vi "SubPanel_DataCollection_Rev11_v5.vi"(0 "DCPowerInformationClusterArray_Input":T6(array[cluster]), 1 "VISAPowerInfoInputArray":T11(array[cluster]), 2 "Run Data SubPanel Input":T10, 3 "RF Block Parameters":T9, 4 "Oscilloscope Info Array":T8(array[cluster]) {"vertical coupling" items=["AC", "DC", "Ground"]}, 6 "New Run?":bool, 7 "error in":errorcluster) -> (10 "data iterating in loop":T2(array[cluster]), 12 "each channel cluster":T2(array[cluster]), 13 "Array of all channels?":dbl[][](array[numeric]), 14 "all channel clusters as a large array":T1(array[cluster]), 16 "data going into the binary file":T3, 20 "DCPowerInformationClusterArray_Output":T6(array[cluster]), 21 "VISAPowerInfoInputOutput":T11(array[cluster]), 22 "Run Data SubPanel Output":T10, 23 "RF Block Parameters Output":T9, 24 "Oscilloscope Info Array Output":T8(array[cluster]) {"vertical coupling" items=["AC", "DC", "Ground"]}, 25 "Reinitialize?":bool, 26 "Data Was Collected?":bool, 27 "error out":errorcluster)   [LabVIEW 2019]
uses:
  Controls/QueueDataControl.ctl
  Controls/DataBlockControl.ctl
  Controls/QueueDataControl_V2.ctl
  <vilib>/Analysis/NI_AALBase.lvlib
  Controls/QueueDataControl_V3.ctl
  <vilib>/Analysis/1siggen.llb/Ramp Pattern by Delta.vi
  <vilib>/Utility/file.llb/Write Delimited Spreadsheet (DBL).vi
  Controls/RFBlockControl.ctl
  <instrlib>/niScope/Controls/niScope vertical coupling.ctl
panel:
  out "supplemental datafile concatenated":i32[](array[numeric])
  out "supplemental datafile array":i32[][](array[numeric])
  out "supplemental datafile":i32[](array[numeric])
  out "datafile in array":T4[][](array[typedef])
  out "datafile in concatenation":T4[](array[typedef])
  out "datafile in loop":T4[](array[typedef])
  out "output cluster 2":T5
  out "Array":dbl[][][](array[numeric])
  out "DCPowerInformationClusterArray_Input 2":T6(array[cluster])
  out "Exiting":bool
  out "output cluster":T5
  out "Full Run Information":string
  out "Ready For Next Run?":bool
  in  "Next Run":bool
  out "Latchup Output Data":dbl[][](array[numeric])
  out "Recording Data":bool
  out "Current 2":waveform(dbl)[](graph)
  out "Voltage 2":waveform(dbl)[](graph)
  out "Current":waveform(dbl)[](graph)
  out "Voltage":waveform(dbl)[](graph)
  in  "End Collecting":bool
  in  "Record Data Toggle":bool
  out "error of collection":errorcluster
  in  "force exit SubVI":bool
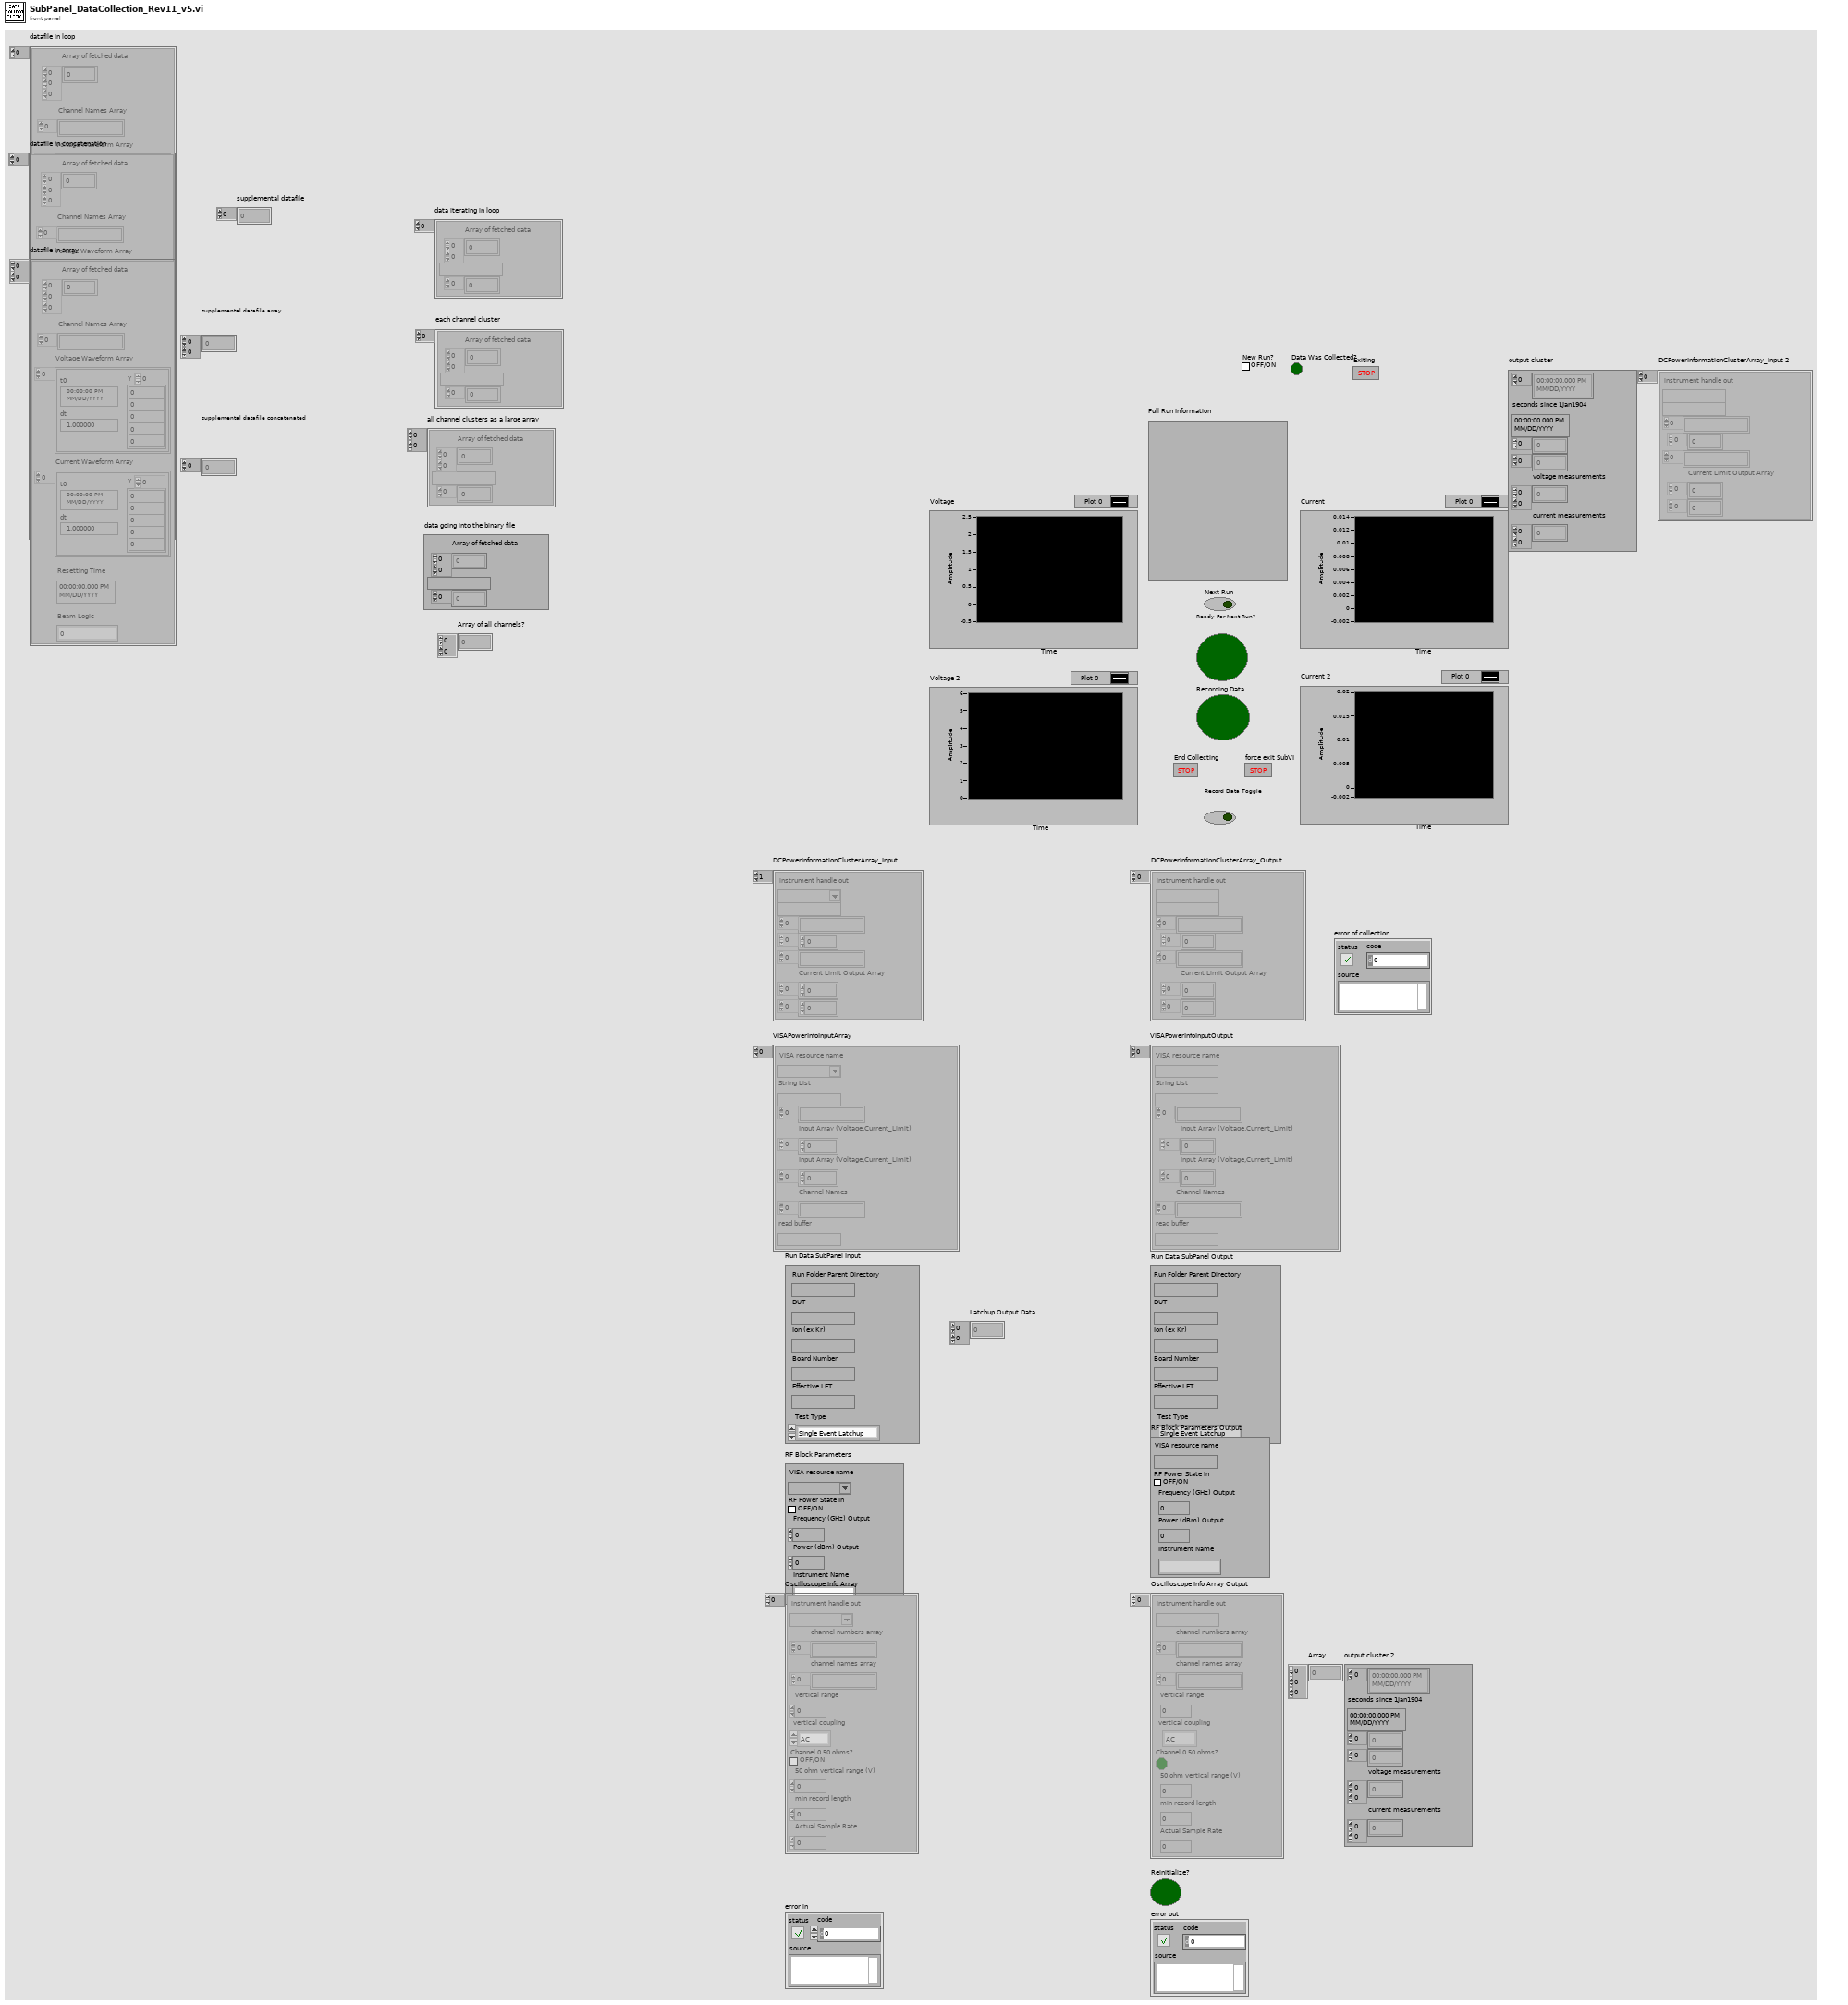
[diagram p1: front panel]
types:
  T1 = cluster{"Array of fetched data":dbl[][], string, i32[]}[][]
  T2 = cluster{"Array of fetched data":dbl[][], string, i32[]}[]
  T3 = cluster{"Array of fetched data":dbl[][], string, i32[]}
  T4 = typedef "QueueDataControl_V3.ctl" = cluster{"Array of fetched data":dbl[][][], "Channel Names Array":string[], "Voltage Waveform Array":waveform(dbl)[], "Current Waveform Array":waveform(dbl)[], "Resetting Time":timestamp, "Beam Logic":dbl}
  T5 = cluster{timestamp[], "seconds since 1Jan1904":timestamp, dbl[], i32[], "voltage measurements":dbl[][], "current measurements":dbl[][]}
  T6 = cluster{"instrument handle out":refnum<k15>, string, string[], dbl[], string[], "Current Limit Output Array":dbl[], dbl[]}[]
  T7 = typedef "niScope vertical coupling.ctl" = i32
  T8 = cluster{"instrument handle out":refnum<k15>, "channel numbers array":string[], "channel names array":string[], "vertical range":dbl, "vertical coupling":T7, "Channel 0 50 ohms?":bool, "50 ohm vertical range (V)":dbl, "min record length":i32, "Actual Sample Rate":dbl}[]
  T9 = typedef "RFBlockControl.ctl" = cluster{"VISA resource name":refnum<visa-resource-name>, "RF Power State In":bool, "Frequency (GHz) Output":dbl, "Power (dBm) Output":dbl, "Instrument Name":string}
  T10 = typedef "DataBlockControl.ctl" = cluster{"Run Folder Parent Directory":path, "DUT":string, "Ion (ex Kr)":string, "Board Number":string, "Effective LET":string, "Test Type":enum16{"Single Event Latchup", "Single Event Transient", "Single Event Upset"}}
  T11 = cluster{"VISA resource name":refnum<visa-resource-name>, "String List":string, string[], "Input Array (Voltage,Current_Limit)":dbl[], "Input Array (Voltage,Current_Limit)":dbl[], "Channel Names":string[], "read buffer":string}[]
  T12 = typedef "QueueDataControl_V2.ctl" = cluster{"Time Stamp Array":timestamp[], "Initial Time":timestamp, "dt measurement array":dbl[], "samples per capture":i32[], "voltage measurements":dbl[][], "current measurements":dbl[][]}
  T13 = cluster{"IVI Refnum out":refnum<k15>, string, "voltage level channel 23":dbl, "Channel Name 23":string, "Current Limit":dbl, "Measure Record dt":dbl, string, "Current Threshold Reset Value Array":dbl, "Mitigation Channel":bool}[]
  T14 = typedef "QueueDataControl.ctl" = cluster{"Rolling Timer":timestamp, "Initial Time":timestamp, "dt between samples":dbl[], "number of samples per fetch":i32[], "voltage measurements":dbl[][], "current measurements":dbl[][]}
  T15 = enum16{"big-endian, network order", "native, host order", "little-endian"}
  T16 = enum16{"open", "replace", "create", "open or create", "replace or create", "replace or create with confirmation"}
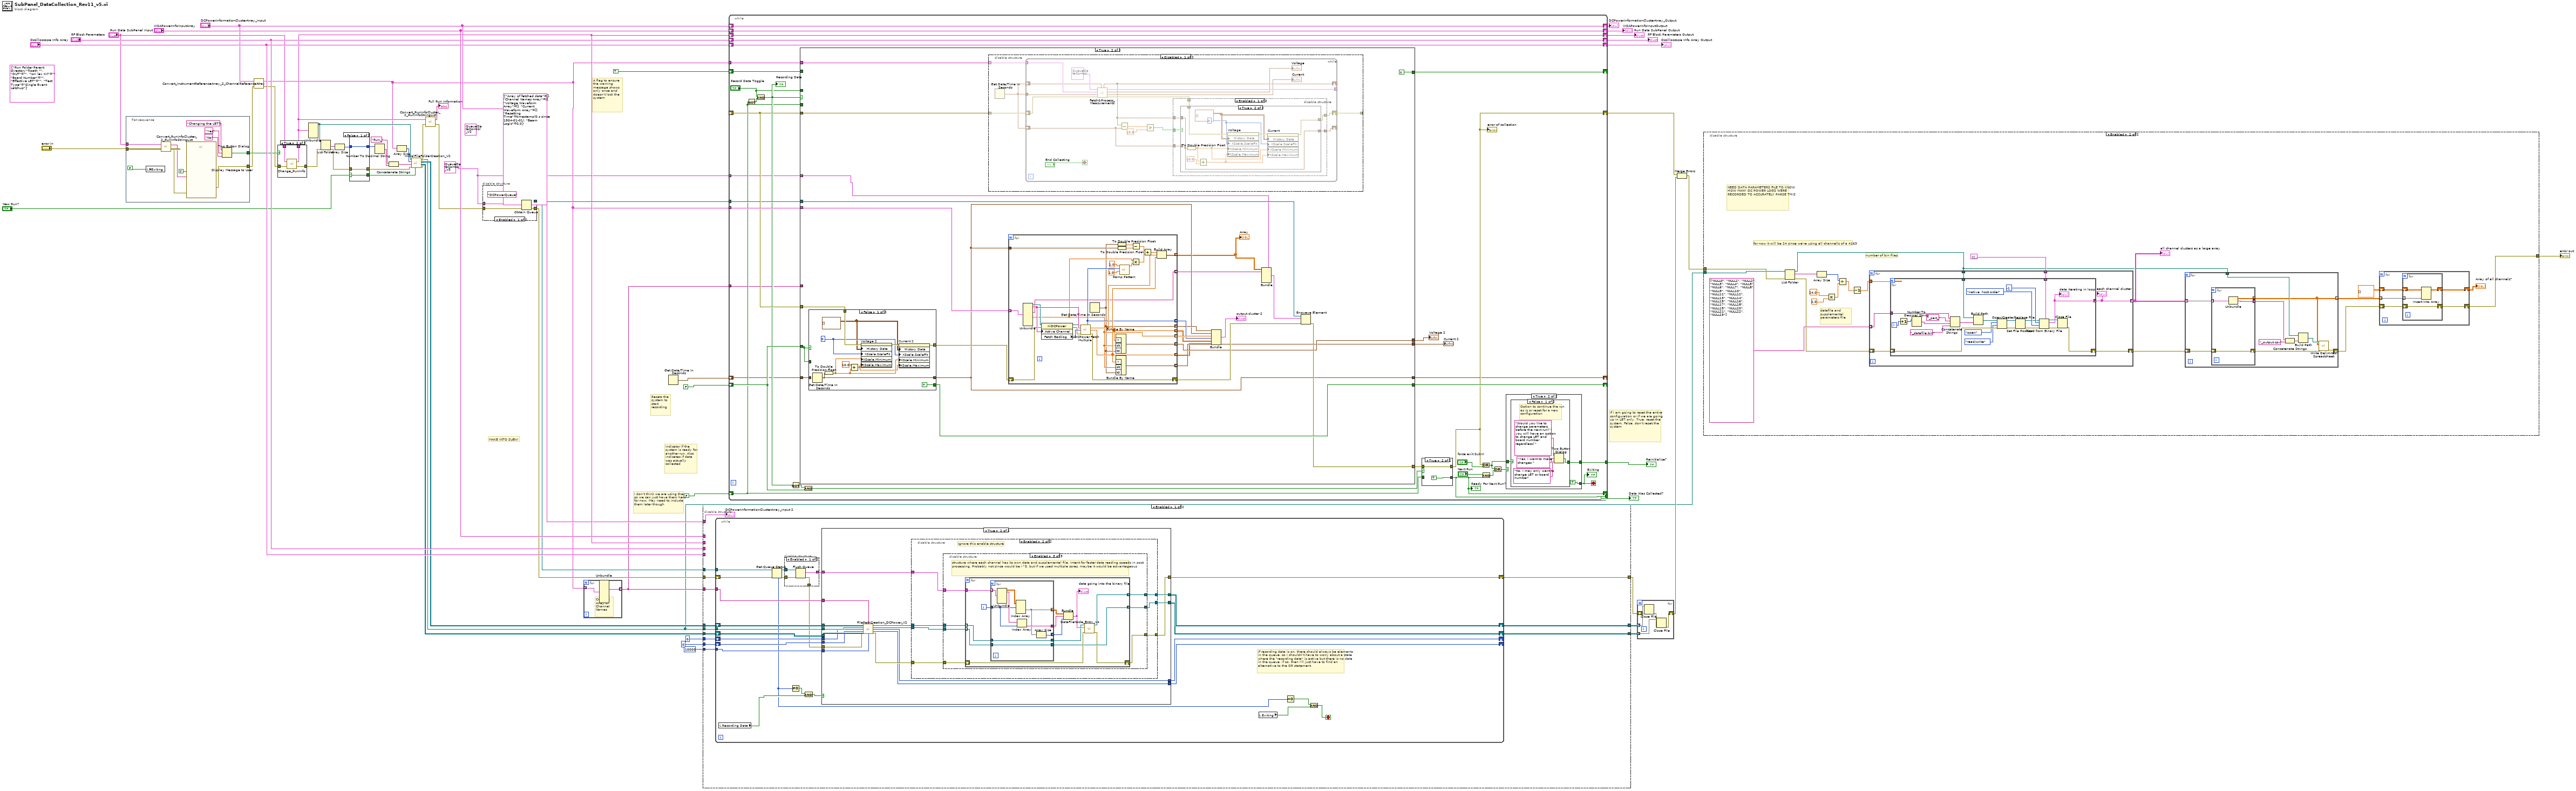
[diagram p0: block diagram]
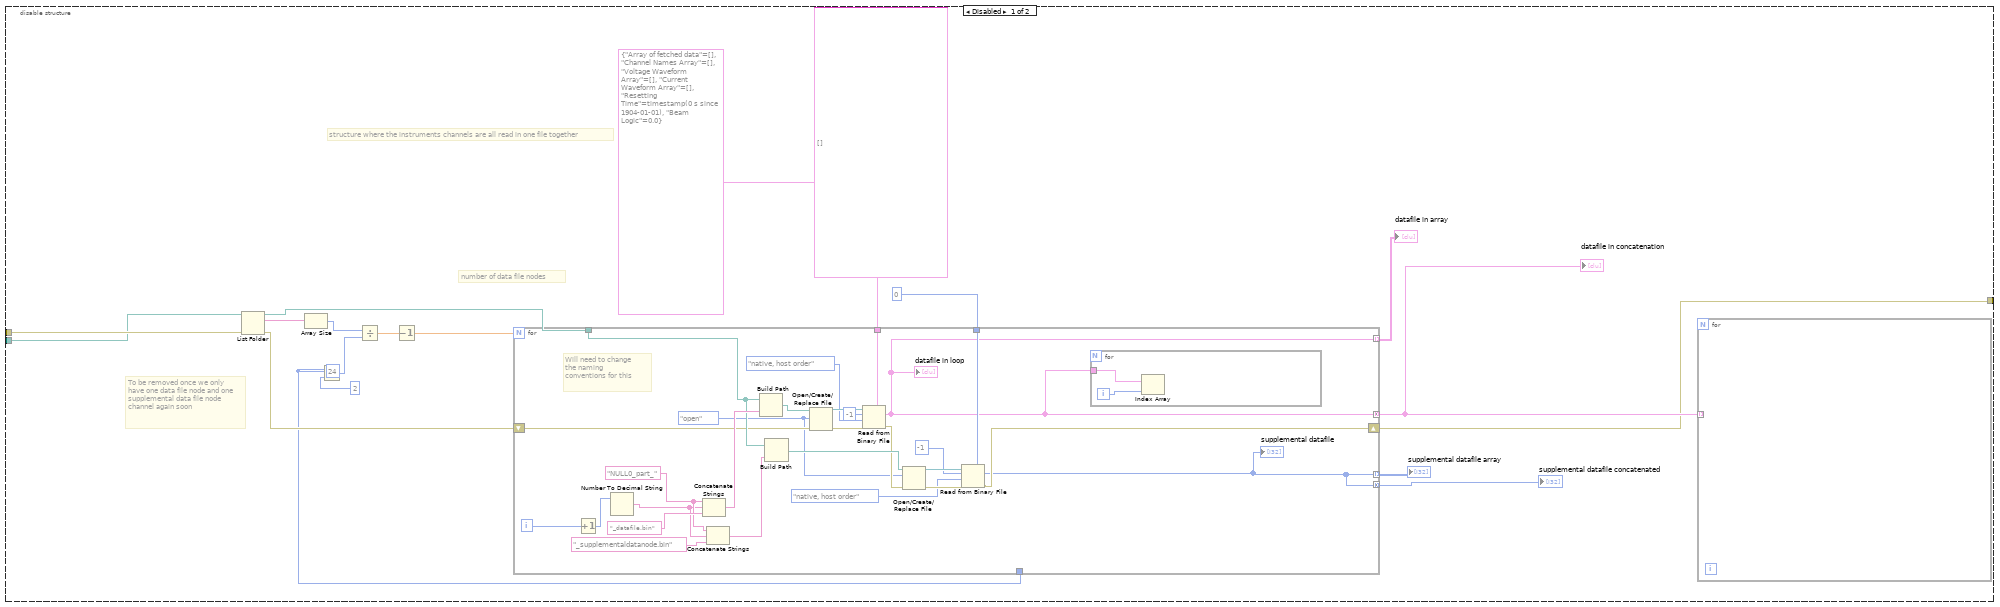
[diagram p2: hidden frame]
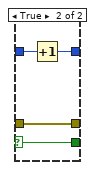
[diagram p3: hidden frame]
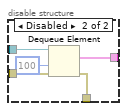
[diagram p6: hidden frame]
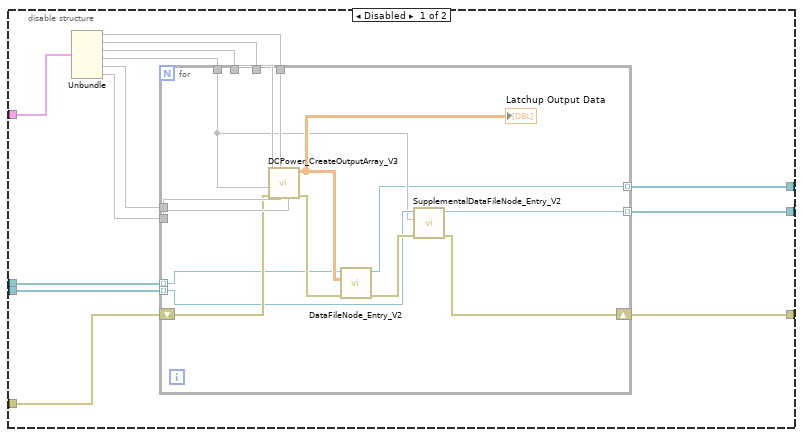
[diagram p8: hidden frame]
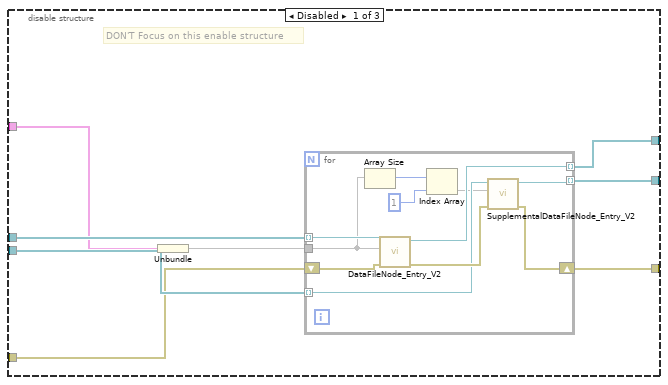
[diagram p9: hidden frame]
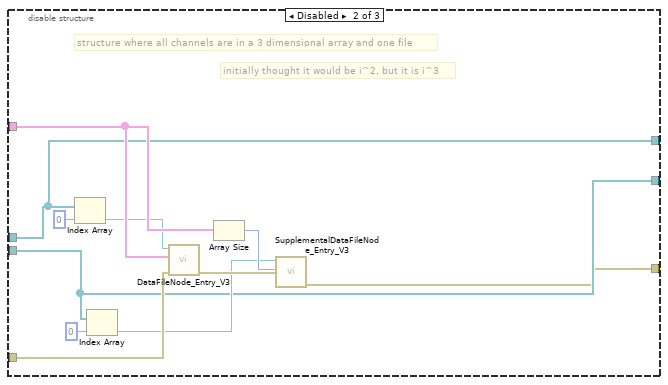
[diagram p10: hidden frame]
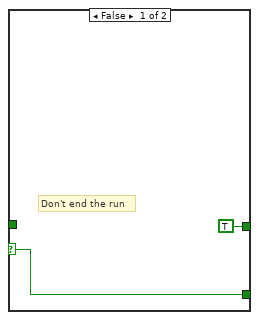
[diagram p12: hidden frame]
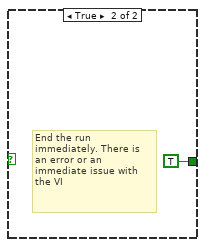
[diagram p13: hidden frame]
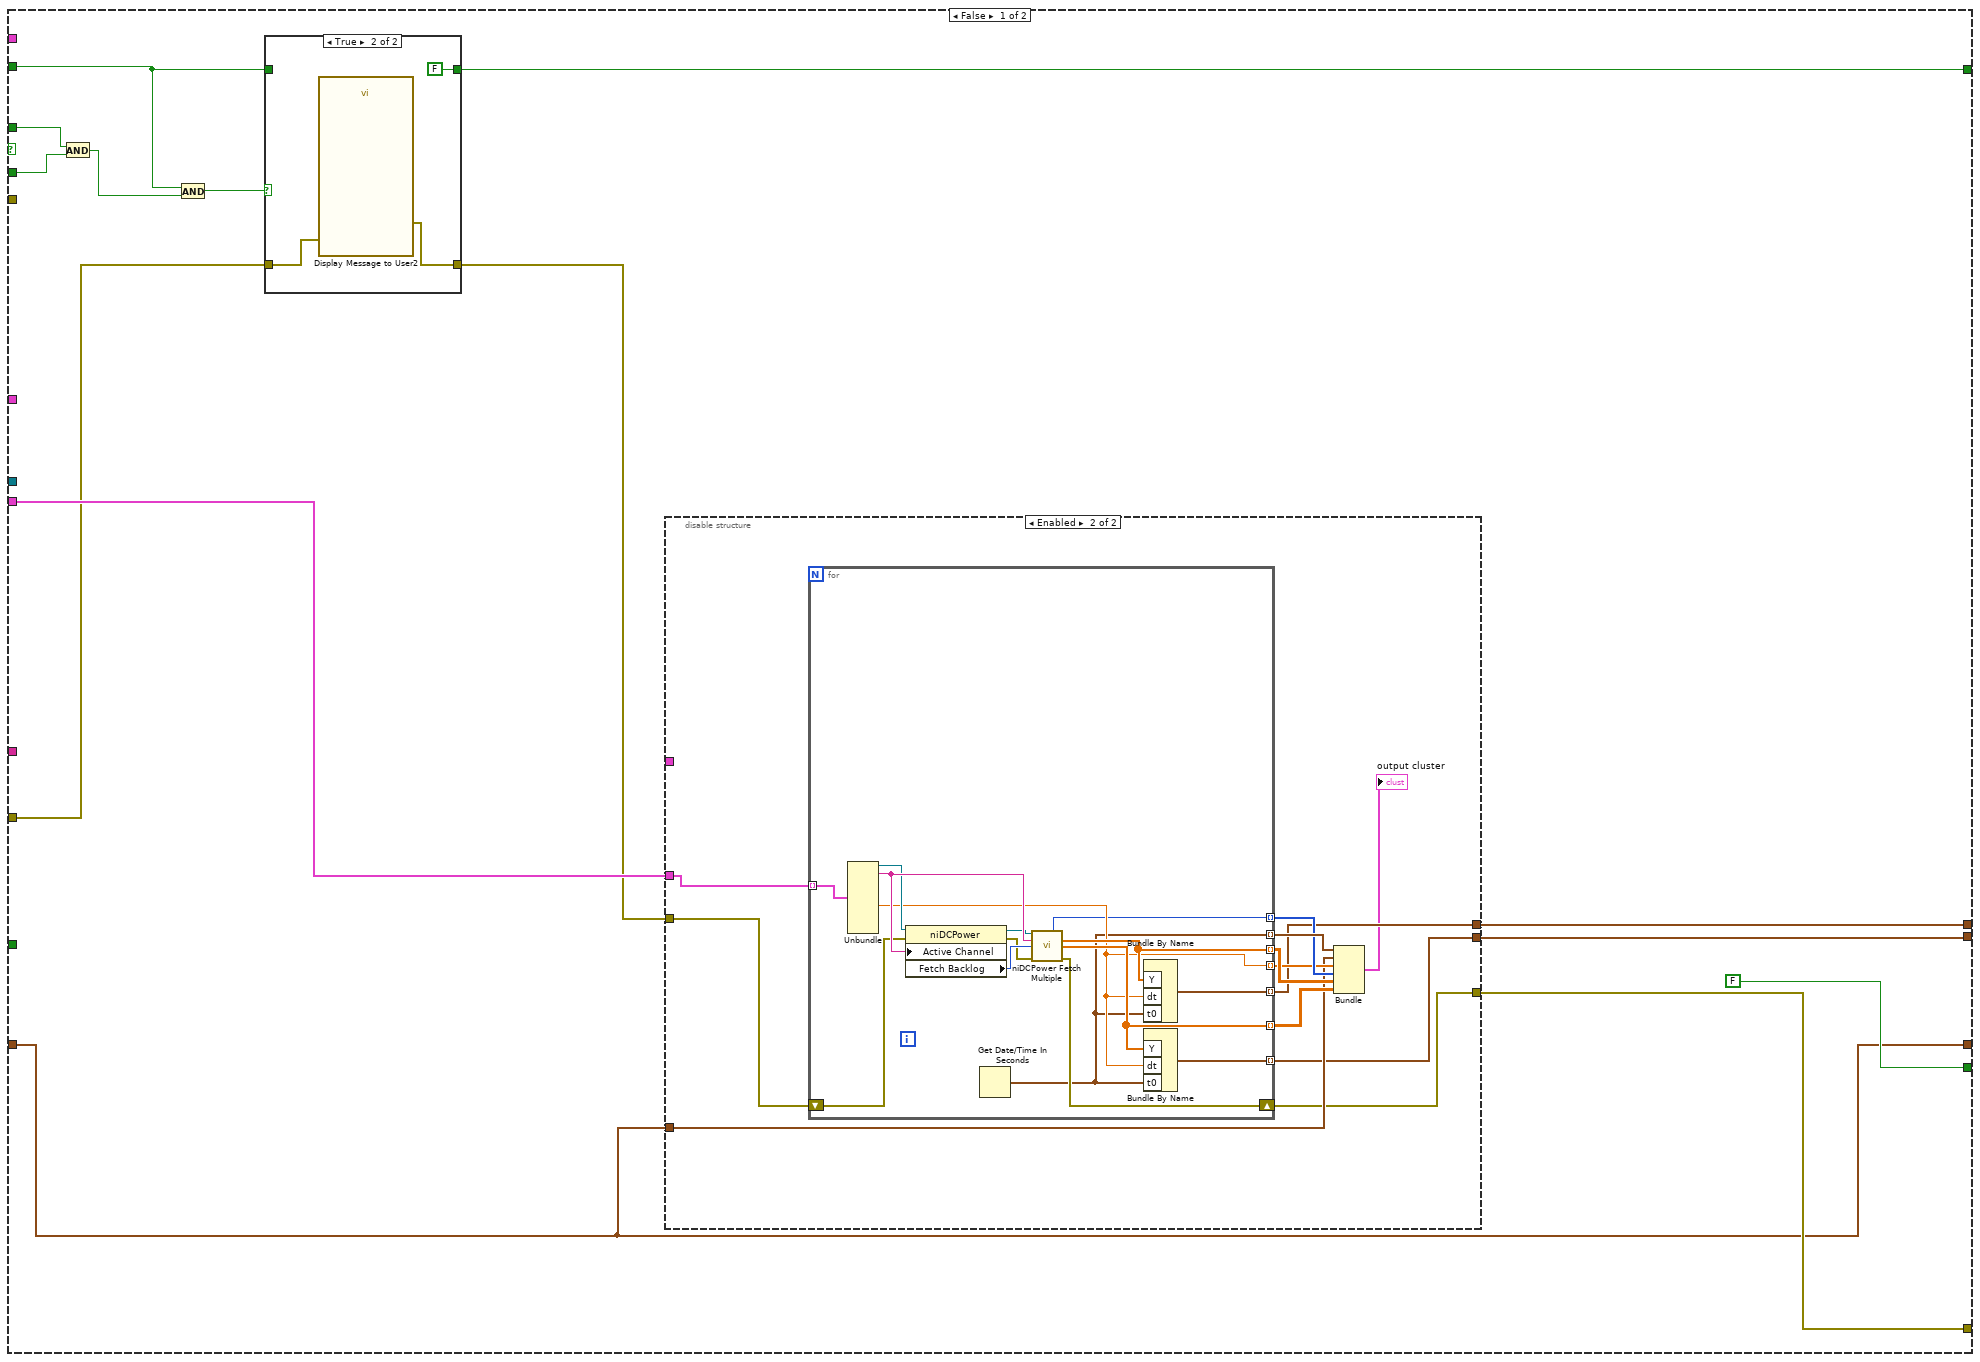
[diagram p15: hidden frame]
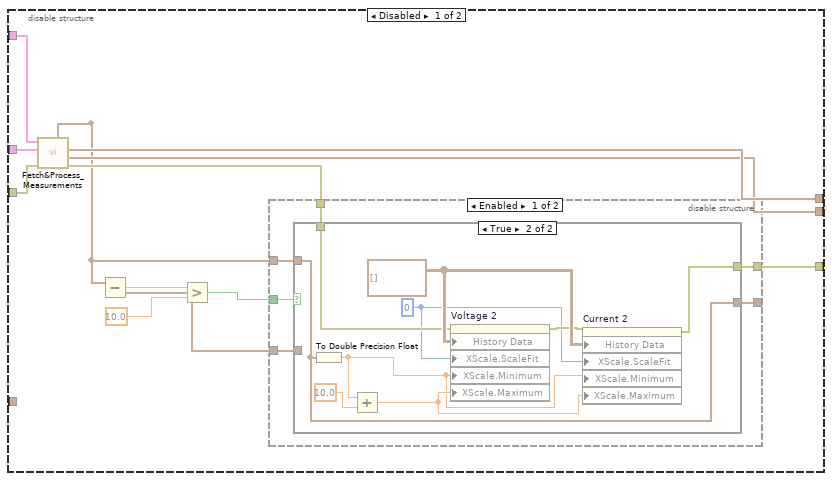
[diagram p16: hidden frame]
diagram:
  w8 = T4 {"Array of fetched data"=[], "Channel Names Array"=[], "Voltage Waveform Array"=[], "Current Waveform Array"=[], "Resetting Time"=timestamp(0 s since 1904-01-01), "Beam Logic"=0.0} ("DCPower Queue Data Double Array Format")
  (unwired) T4 {"Array of fetched data"=[], "Channel Names Array"=[], "Voltage Waveform Array"=[], "Current Waveform Array"=[], "Resetting Time"=timestamp(0 s since 1904-01-01), "Beam Logic"=0.0} ("DCPower Double Array Queue")
  (unwired) T12 {"Time Stamp Array"=[], "Initial Time"=timestamp(0 s since 1904-01-01), "dt measurement array"=[], "samples per capture"=[], "voltage measurements"=[], "current measurements"=[]} ("DCPowerDataQueueControl_V2")
  (unwired) T10 {"Run Folder Parent Directory"=path "", "DUT"="", "Ion (ex Kr)"="", "Board Number"="", "Effective LET"="", "Test Type"=enum."Single Event Latchup"} ("Run Data Configuration")
  # "I don't think we are using these so we can just have them here for now. May need to include them later though"
  # "Indicator if the system is ready for another run. Also indicates if data was actually collected"
  # "Resets the system to start recording"
  # "A flag to ensure the warning message shows only once and doesn't lock the system"
  # "If I am going to reset the entire configuration or if we are going up in LET only. True, reset the system. False, don't reset the system"
  # "MAKE INTO SUBVI"
  n1 = flat-sequence {
    tunnel: [w62] -> w31
    tunnel: "error in" -> [w61]
    tunnel: [w66] -> w40
    tunnel: "Run Data SubPanel Input" -> [w59]
    frame #0 {
      n2 = local write "Exiting"(FALSE ("Forced Exit")) -> ()
      n3 = call "Convert_RunInfoCluster_2_RunInfoStringList.vi"("error in"=w61, "Run Data SubPanel Input"=w59) -> ("error output"=w60:errorcluster, "Run Data Output"=w58:string)
      n4 = call "Display Message to User"("error in (no error)"=w60, "Enable"=TRUE, "Message"=w58) -> ("error out"=w62:errorcluster)  [unwired: 7 in, 1 out]
      n5 = Two Button Dialog(message="Changing the LET?", 1:"No" ("F button name (\"Cancel\")"), 2:"Yes" ("T button name (\"OK\")")) -> (T button?=w66:bool)
    }
  }
  n6 = call "Convert_InstrumentReferenceArray_2_ChannelReferenceArray.vi"("error in (no error)"=w31, "DCPowerInformationClusterArray_Input"="DCPowerInformationClusterArray_Input") -> ("error out"=w29:errorcluster, "DCPowerInformationArrayOutput_byChannel"=w14:T13)
  n7 = case shown="True" w40 {
    tunnel: "Run Data SubPanel Input" -> [w68 w72]
    tunnel: [w68 w71] -> w36
    tunnel: [w67 w70] -> w33
    tunnel: w29 -> [w67 w69]
    frame False {
    }
    frame True {
      n8 = call "Change_RunInfo.vi"("error in (no error)"=w69, "Run Data SubPanel in"=w72) -> ("error out"=w70:errorcluster, "Run Data SubPanel out"=w71:T10)
    }
  }
  n9 = Unbundle(w36) -> ("Run Folder Parent Directory"=w34:path)  [unwired: 5 out]
  n10 = List Folder(path=w34, error in=w33) -> (folder names=w35:string[], error out=w15:errorcluster)  [unwired: 2 in, 2 out]
  n11 = Array Size(array=w35) -> (size(s)=w18:i32)
  n12 = case shown="False" "New Run?" {
    selector: "New Run?" -> [w74 w77]
    tunnel: [w75 w79] -> w19
    tunnel: w18 -> [w75 w78]
    tunnel: [w74 w77] -> w17
    tunnel: [w73 w76] -> w16
    tunnel: w15 -> [w73 w76]
    frame False {
    }
    frame True {
      n13 = Increment(x=w78) -> (x+1=w79:i32)
    }
  }
  n14 = Number To Decimal String(number=w19) -> (decimal integer string=w23:string)  [unwired: 1 in]
  n15 = Concatenate Strings("Run_", w23) -> (w32:string)
  n16 = Array Size(array=w14) -> (size(s)=w13:i32)
  n17 = call "InitialFileFolderCreation_V2.vi"("New Run?"=w17, "error in (no error)"=w16, "Run Number"=w32, "Subfolders&NumChannelsRecorded"=w13, "base path"=w34) -> ("error out"=w12:errorcluster, "SupplementalDataFileReferenceObjectArrayWsubfolders"=w27:refnum<file>[][], "DataFileReferenceObjectArrayWsubfolders"=w28:refnum<file>[][], "created path array"=w2:path[])  [unwired: 3 in]
  n18 = call "Convert_RunInfoCluster_2_RunInfoStringList.vi"("error in"=w12, "Run Data SubPanel Input"=w36) -> ("error output"=w11:errorcluster, "Run Data Output"=→"Full Run Information":string)
  n19 = disable-structure shown="Enabled" {
    disable-tunnel: w11 -> [w83 w85]
    disable-tunnel: [w82 w85] -> w45
    disable-tunnel: [w81 _] -> w46
    disable-tunnel: w8 -> [w80 _]
    frame Enabled {
      n20 = Obtain Queue(name (unnamed)="DCPowerQueue", element data type=w80, error in (no error)=w83) -> (queue out=w81:refnum<queue>, error out=w82:errorcluster)  [unwired: 2 in, 1 out]
    }
    frame Disabled {
    }
  }
  n21 = for {
    tunnel: w14 -> [w87] mode=indexing
    tunnel: [w86] -> w9 mode=indexing
    # "Creating Array of Channel Names"
    n22 = Unbundle(w87) -> ("Channel Name 23"=w86:string)  [unwired: 8 out]
  }
  n23 = Get Date/Time In Seconds() -> (seconds since 1Jan1904=w37:timestamp)
  n24 = disable-structure shown="Enabled" {
    disable-tunnel: "DCPowerInformationClusterArray_Input" -> [w91 _]
    disable-tunnel: "VISAPowerInfoInputArray" -> [_ _]
    disable-tunnel: w36 -> [_ _]
    disable-tunnel: "RF Block Parameters" -> [_ _]
    disable-tunnel: "Oscilloscope Info Array" -> [_ _]
    disable-tunnel: w46 -> [w100 _]
    disable-tunnel: w45 -> [w99 _]
    disable-tunnel: w9 -> [w98 _]
    disable-tunnel: w2 -> [w97 _]
    disable-tunnel: w28 -> [w96 _]
    disable-tunnel: w27 -> [w95 _]
    disable-tunnel: 0 ("binary file indexor in") -> [w94 _]
    disable-tunnel: 0 ("binary file indexor in") -> [w93 _]
    disable-tunnel: 10000 ("binary file indexor in") -> [w92 _]
    disable-tunnel: [w90 _] -> w5
    disable-tunnel: [w89 _] -> w7
    disable-tunnel: [w88 _] -> w6
    frame Enabled {
      n25 = while {
        tunnel: w100 -> [w125]
        shift-right: [w112] -> w90
        shift-left: w99 -> [w124]
        tunnel: w97 -> [w121]
        shift-right: [w114] -> w89
        shift-left: w96 -> [w122]
        shift-right: [w113] -> w88
        shift-left: w95 -> [w120]
        shift-right: [w116] -> _
        shift-left: w94 -> [w119]
        shift-right: [w115] -> _
        shift-left: w93 -> [w118]
        tunnel: w92 -> [w117]
        tunnel: w98 -> [w123]
        stop <- w109 stop-if-true
        # "If recording data is on, there should always be elements in the queue, so I shouldn't have to worry about a state where the \"recording data\" is active but there is no data in the queue, if so, then I'll just have to find an alternative to the OR statement"
        n26 = local read "Recording Data"() -> (w102:bool)
        n27 = Get Queue Status(queue=w125, error in (no error)=w124) -> (queue out=w106:refnum<queue>, error out=w107:errorcluster, # elements in queue=w101:i32)  [unwired: 1 in, 5 out]
        n28 = disable-structure shown="Enabled" {
          disable-tunnel: [w129 w131] -> w108
          disable-tunnel: w107 -> [w128 w133]
          disable-tunnel: w106 -> [w127 w134]
          disable-tunnel: [w126 w130] -> w105
          frame Enabled {
            n29 = Flush Queue(queue=w127, error in (no error)=w128) -> (remaining elements=w126:T4[], error out=w129:errorcluster)  [unwired: 1 out]
          }
          frame Disabled {
            n30 = Dequeue Element(queue=w134, timeout in ms (-1)=100, error in (no error)=w133) -> (element=w130:T4, error out=w131:errorcluster)  [unwired: 2 out]
          }
        }
        n31 = Not Equal To 0?(x=w101) -> (x != 0?=w104:bool)
        n32 = And(x=w104, y=w102) -> (x .and. y?=w103:bool)
        n33 = case shown="True" w103 {
          tunnel: w105 -> [_ w156]
          tunnel: w108 -> [w137 w149]
          tunnel: w123 -> [_ w155]
          tunnel: w122 -> [w138 w154]
          tunnel: w121 -> [_ w153]
          tunnel: w120 -> [w139 w152]
          tunnel: w119 -> [w136 w151]
          tunnel: w118 -> [w135 w148]
          tunnel: w117 -> [_ w147]
          tunnel: [w136 w146] -> w116
          tunnel: [w135 w145] -> w115
          tunnel: [w138 w142] -> w114
          tunnel: [w139 w141] -> w113
          tunnel: [w137 w140] -> w112
          frame False {
          }
          frame True {
            n34 = call "FilePathCreation_DCPower_V2.vi"("binary file input reference array 1"=w154, "Channel Name Input array"=w155, "data output directory folder"=w153, "binary file indexor in"=w151, "Reset counter in"=w148, "error in (no error)"=w149, "binary file input reference array 2"=w152, "reset threshold"=w147) -> ("binary file output reference array"=w144:refnum<file>[], "binary file output reference array 2"=w143:refnum<file>[], "binary file indexor out"=w146:i32, "reset counter out"=w145:i32, "error out"=w150:errorcluster)  [unwired: 3 in]
            n35 = disable-structure shown="Enabled" {
              disable-tunnel: w156 -> [w169 w185]
              disable-tunnel: w150 -> [w168 w189]
              disable-tunnel: w144 -> [w167 w191]
              disable-tunnel: w143 -> [w166 w190]
              disable-tunnel: [w165 w188] -> w142
              disable-tunnel: [w164 w187] -> w141
              disable-tunnel: [w163 w186] -> w140
              frame Disabled {
                n36 = Unbundle(w169) -> (w157, w158, w162, w161, w160, w159)
                n37 = for {
                  tunnel: w162 -> [w182]
                  tunnel: w161 -> [w172]
                  tunnel: w160 -> [w181]
                  tunnel: w159 -> [w180]
                  tunnel: w158 -> [w183]
                  tunnel: w157 -> [w184]
                  shift-right: [w174] -> w163
                  shift-left: w168 -> [w179]
                  tunnel: w167 -> [w176] mode=indexing
                  tunnel: w166 -> [w173] mode=indexing
                  tunnel: [w171] -> w165 mode=indexing
                  tunnel: [w170] -> w164 mode=indexing
                  n38 = call "DCPower_CreateOutputArray_V3.vi"("current measurements"=w180, "voltage measurements"=w181, "Time Stamp Array"=w184, "error in"=w179, "actual count"=w172, "Measure Record dt"=w182, "Initial Time"=w183) -> ("error out"=w178:errorcluster, "Data Output Array"=w177:dbl[][])  [unwired: 3 in]
                  "Latchup Output Data" <- w177
                  n39 = call "DataFileNode_Entry_V2.vi"("error in (no error)"=w178, "Data Output Array"=w177, "Byte Stream File in"=w176) -> ("error out"=w175:errorcluster, "Byte Stream File out"=w171:refnum<file>)  [unwired: 7 in]
                  n40 = call "SupplementalDataFileNode_Entry_V2.vi"("error in (no error)"=w175, "actual count"=w172, "Byte Stream File in"=w173) -> ("error out"=w174:errorcluster, "Byte Stream File out"=w170:refnum<file>)  [unwired: 7 in]
                }
              }
              frame Enabled {
                # "Ignore this enable structure"
                n41 = disable-structure shown="Enabled" {
                  disable-tunnel: w191 -> [w199 w213 w228]
                  disable-tunnel: w190 -> [w198 w212 w227]
                  disable-tunnel: w189 -> [w197 w221 w225]
                  disable-tunnel: [w196 w213 w223] -> w188
                  disable-tunnel: [w195 w212 w222] -> w187
                  disable-tunnel: [w194 w211 w226] -> w186
                  disable-tunnel: w185 -> [w193 w218 w224]
                  frame Disabled {
                    # "DON'T Focus on this enable structure"
                    n42 = Unbundle(w193) -> (w192)
                    n43 = for {
                      tunnel: w192 -> [w207]
                      tunnel: w199 -> [w209] mode=indexing
                      tunnel: w198 -> [w208] mode=indexing
                      tunnel: [w205] -> w196 mode=indexing
                      tunnel: [w204] -> w195 mode=indexing
                      shift-right: [w203] -> w194
                      shift-left: w197 -> [w206]
                      n44 = Array Size(array=w207) -> (size(s)=w202:i32)
                      n45 = call "DataFileNode_Entry_V2.vi"("error in (no error)"=w206, "Data Output Array"=w207, "Byte Stream File in"=w209) -> ("error out"=w210:errorcluster, "Byte Stream File out"=w205:refnum<file>)  [unwired: 7 in]
                      n46 = Index Array(array=w202, index=1) -> (element=w200)
                      n47 = call "SupplementalDataFileNode_Entry_V2.vi"("error in (no error)"=w210, "actual count"=w200, "Byte Stream File in"=w208) -> ("error out"=w203:errorcluster, "Byte Stream File out"=w204:refnum<file>)  [unwired: 7 in]
                    }
                  }
                  frame Disabled {
                    # "initially thought it would be i^2, but it is i^3"
                    # "structure where all channels are in a 3 dimensional array and one file"
                    n48 = Index Array(array=w213, index=0) -> (element=w214:refnum<file>)
                    n49 = Index Array(array=w212, index=0) -> (element=w215:refnum<file>)
                    n50 = call "DataFileNode_Entry_V3.vi"("error in (no error)"=w221, "remaining elements"=w218, "Byte Stream File in"=w214) -> ("error out"=w220:errorcluster)  [unwired: 7 in, 1 out]
                    n51 = Array Size(array=w218) -> (size(s)=w219:i32)
                    n52 = call "SupplementalDataFileNode_Entry_V3.vi"("error in (no error)"=w220, "actual count"=w219, "Byte Stream File in"=w215) -> ("error out"=w211:errorcluster)  [unwired: 7 in, 1 out]
                  }
                  frame Enabled {
                    # "structure where each channel has its own data and supplemental file. Intent for faster data reading speeds in post processing. Probably not since would be i^3, but if we used multiple cores, maybe it would be advantageous"
                    n53 = for {
                      tunnel: w228 -> [w236] mode=indexing
                      tunnel: w227 -> [w237] mode=indexing
                      shift-right: [w229] -> w226
                      shift-left: w225 -> [w232]
                      tunnel: w224 -> [w241]
                      tunnel: [w231] -> w223 mode=indexing
                      tunnel: [w230] -> w222 mode=indexing
                      i -> [w240]
                      n54 = for {
                        tunnel: w241 -> [w250] mode=indexing
                        tunnel: w240 -> [w247]
                        tunnel: [w243] -> w239 mode=concatenating
                        tunnel: [w246] -> w238
                        tunnel: w237 -> [w244]
                        tunnel: w236 -> [w245]
                        tunnel: [w245] -> w233
                        tunnel: [w244] -> w230
                        tunnel: [w242] -> w235 mode=concatenating
                        n55 = Unbundle(w250) -> ("Array of fetched data"=w249:dbl[][][], "Channel Names Array"=w248:string[])  [unwired: 4 out]
                        n56 = Index Array(array=w249, index (dim 0)=w247) -> (element=w243:dbl[][])  [unwired: 2 in]
                        n57 = Index Array(array=w248, index=w247) -> (element=w246:string)
                        n58 = Array Size(array=w243) -> (size(s)=w242:i32[])
                      }
                      n59 = Bundle("Array of fetched data"=w239, w238, w235) -> (w234:T3)  [unwired: 1 in]
                      "data going into the binary file" <- w234
                      n60 = call "DataFileNode_Entry_V4.vi"("error in (no error)"=w232, "Queued Elements"=w234, "Byte Stream File in"=w233) -> ("error out"=w229:errorcluster, "Byte Stream File out"=w231:refnum<file>)  [unwired: 7 in]
                    }
                  }
                }
              }
            }
          }
        }
        n61 = local read "Exiting"() -> (w111:bool)
        n62 = Equal To 0?(x=w101) -> (x = 0?=w110:bool)
        n63 = And(x=w110, y=w111) -> (x .and. y?=w109:bool)
      }
      "DCPowerInformationClusterArray_Input 2" <- w91
    }
    frame Disabled {
    }
  }
  n64 = while {
    shift-right: [w281] -> w55
    shift-left: "DCPowerInformationClusterArray_Input" -> [w281]
    shift-right: [w285] -> w54
    shift-left: "VISAPowerInfoInputArray" -> [w285]
    shift-right: [w284] -> w53
    shift-left: w36 -> [w284]
    shift-right: [w283] -> w52
    shift-left: "RF Block Parameters" -> [w283]
    shift-right: [w282] -> w51
    shift-left: "Oscilloscope Info Array" -> [w282]
    shift-right: [w265] -> w10
    shift-left: _ -> [w278]
    tunnel: w14 -> [w280]
    tunnel: w14 -> [w279]
    shift-right: [w275] -> _
    shift-left: FALSE -> [w272]
    tunnel: w46 -> [w274]
    shift-right: [w254] -> _
    shift-left: FALSE -> [w259]
    tunnel: [w263] -> w44
    shift-right: [w257] -> _
    shift-left: TRUE ("x .and. y?") -> [w258]
    shift-right: [w255] -> _
    shift-left: w37 -> [w256]
    tunnel: [w254] -> w21
    tunnel: w9 -> [w252]
    tunnel: w8 -> [w251]
    stop <- w253 stop-if-true
    n65 = Not(x=w259) -> (.not. x?=w261:bool)
    n66 = And(x="Record Data Toggle", y=w261) -> (x .and. y?=w262:bool)
    "Recording Data" <- w262
    n67 = Not(x=w262) -> (.not. x?=w273:bool)
    n68 = case shown="True" w262 {
      tunnel: w278 -> [_ w403]
      tunnel: w280 -> [_ w402]
      tunnel: w279 -> [w313 w400]
      tunnel: w278 -> [w308 w398]
      tunnel: [w311 w390] -> w277
      tunnel: [w312 w391] -> w276
      tunnel: w272 -> [_ w395]
      tunnel: [FALSE w396] -> w275
      tunnel: w274 -> [_ w394]
      tunnel: [w309 w389] -> w270
      tunnel: "Record Data Toggle" -> [w305 _]
      tunnel: w259 -> [w306 _]
      tunnel: w258 -> [w301 _]
      tunnel: [w302 TRUE] -> w257
      tunnel: w256 -> [w300 w399]
      tunnel: [w300 w383] -> w255
      tunnel: w252 -> [_ _]
      tunnel: w251 -> [_ w380]
      frame False {
        n69 = And(x=w305, y=w306) -> (x .and. y?=w304:bool)
        n70 = And(x=w301, y=w304) -> (x .and. y?=w303:bool)
        n71 = case shown="True" w303 {
          tunnel: [w375 w377] -> w307
          tunnel: w308 -> [w375 w378]
          tunnel: [w374 FALSE] -> w302
          tunnel: w301 -> [w374 _]
          frame False {
          }
          frame True {
            n72 = call "Display Message to User2"("error in (no error)"=w378) -> ("error out"=w377:errorcluster)  [unwired: 9 in, 1 out]
          }
        }
        n73 = disable-structure shown="Enabled" {
          disable-tunnel: w313 -> [w323 w353]
          disable-tunnel: _ -> [w322 _]
          disable-tunnel: [w318 w351] -> w312
          disable-tunnel: [w317 w350] -> w311
          disable-tunnel: [w315 w349] -> w309
          disable-tunnel: w307 -> [w314 w348]
          disable-tunnel: w300 -> [_ w352]
          frame Disabled {
            n74 = call "Fetch&Process_Measurements.vi"("error in (no error)"=w314, "DCPowerInformation_byChannel"=w323, "Queue Data Parameters in"=w322) -> ("error out"=w324:errorcluster, "Current Measurement"=w317:waveform(dbl)[], "Voltage Measurement"=w318:waveform(dbl)[], "Rolling Timer Output"=w316:timestamp, "Rolling Timer Input"=w321:timestamp)  [unwired: 3 in, 1 out]
            n75 = Subtract(x=w316, y=w319) -> (x-y=w326:dbl)
            n76 = Greater?(x=w326, y=10.0) -> (0:w325:bool)
            n77 = disable-structure shown="Enabled" {
              disable-tunnel: w325 -> [w333 _]
              disable-tunnel: w324 -> [w332 w346]
              disable-tunnel: [w331 w346] -> w315
              disable-tunnel: [w330 w345] -> w320
              disable-tunnel: w316 -> [w329 w345]
              disable-tunnel: [w328 _] -> w319
              frame Enabled {
                n78 = case shown="True" w333 {
                  tunnel: w332 -> [w335 w341]
                  tunnel: [w335 w339] -> w331
                  tunnel: [w334 w343] -> w330
                  tunnel: w329 -> [_ w343]
                  tunnel: w328 -> [w334 _]
                  frame False {
                  }
                  frame True {
                    w338 = u8 0 ("X Scale.Scale Fit")
                    w342 = waveform(dbl)[][] [] ("History Data")
                    n79 = To Double Precision Float(number=w343) -> (double precision float=w336:dbl)
                    n80 = Add(x=w336, y=10.0) -> (x+y=w337:dbl)
                    n81 = property on="Voltage 2" class="WFChart (strict)"(error in=w341, "History Data"=w342, "XScale.ScaleFit"=w338, "XScale.Minimum"=w336, "XScale.Maximum"=w337) -> (error out=w340:errorcluster)  [unwired: 1 in, 1 out]
                    n82 = property on="Current 2" class="WFChart (strict)"(error in=w340, "History Data"=w342, "XScale.ScaleFit"=w338, "XScale.Minimum"=w336, "XScale.Maximum"=w337) -> (error out=w339:errorcluster)  [unwired: 1 in, 1 out]
                  }
                }
              }
              frame Disabled {
              }
            }
          }
          frame Enabled {
            n83 = for {
              tunnel: w353 -> [w373] mode=indexing
              tunnel: [w366] -> w351 mode=indexing
              tunnel: [w365] -> w350 mode=indexing
              tunnel: [w360] -> w355 mode=indexing
              tunnel: [w364] -> w357 mode=indexing
              tunnel: [w363] -> w356 mode=indexing
              tunnel: [w359] -> w358 mode=indexing
              tunnel: [w361] -> w354 mode=indexing
              shift-right: [w362] -> w349
              shift-left: w348 -> [w370]
              n84 = Unbundle(w373) -> ("IVI Refnum out"=w369:refnum<k15>, w372:string, "Measure Record dt"=w361:dbl)  [unwired: 6 out]
              n85 = property class="niDCPower"(reference=w369, error in=w370, "Active Channel"=w372) -> (reference out=w368:refnum<k15>, error out=w367:errorcluster, "Fetch Backlog"=w371:i32)
              n86 = Get Date/Time In Seconds() -> (seconds since 1Jan1904=w359:timestamp)
              n87 = call <instrlib>:"niDCPower Fetch Multiple.vi"("instrument handle"=w368, "channel name"=w372, "count (1)"=w371, "error in (no error)"=w367) -> ("actual count"=w360:i32, "voltage measurements"=w363:dbl[], "current measurements"=w364:dbl[], "error out"=w362:errorcluster)  [unwired: 6 in, 2 out]
              n88 = Bundle By Name("Y"=w363, "dt"=w361, "t0"=w359) -> (w366:waveform(dbl))  [unwired: 1 out]
              n89 = Bundle By Name("Y"=w364, "dt"=w361, "t0"=w359) -> (w365:waveform(dbl))  [unwired: 1 out]
            }
            n90 = Bundle(w358, "seconds since 1Jan1904"=w352, w354, w355, "voltage measurements"=w356, "current measurements"=w357) -> (→"output cluster":T5)  [unwired: 1 in]
          }
        }
      }
      frame True {
        n91 = case shown="False" w395 {
          tunnel: [w434 w442] -> w383
          tunnel: w399 -> [_ w442]
          tunnel: w398 -> [w439 w441]
          tunnel: [w437 w441] -> w397
          tunnel: [TRUE w440] -> w396
          tunnel: w395 -> [_ w440]
          frame False {
            w430 = waveform(dbl)[][] [] ("History Data")
            w435 = u8 0 ("X Scale.Scale Fit")
            n92 = Get Date/Time In Seconds() -> (seconds since 1Jan1904=w434:timestamp)
            n93 = To Double Precision Float(number=w434) -> (double precision float=w431:dbl)
            n94 = Add(x=10.0 ("y"), y=w431) -> (x+y=w433:dbl)
            n95 = property on="Voltage 2" class="WFChart (strict)"(error in=w439, "History Data"=w430, "XScale.ScaleFit"=w435, "XScale.Minimum"=w431, "XScale.Maximum"=w433) -> (error out=w438:errorcluster)  [unwired: 1 in, 1 out]
            n96 = property on="Current 2" class="WFChart (strict)"(error in=w438, "History Data"=w430, "XScale.ScaleFit"=w435, "XScale.Minimum"=w431, "XScale.Maximum"=w433) -> (error out=w437:errorcluster)  [unwired: 1 in, 1 out]
          }
          frame True {
          }
        }
        n97 = disable-structure shown="Disabled" {
          disable-tunnel: w403 -> [w446 _]
          disable-tunnel: w402 -> [w445 _]
          disable-tunnel: [w444 errorcluster {"status"=FALSE, "code"=0, "source"=""} ("error out")] -> _
          frame Disabled {
            n98 = Get Date/Time In Seconds() -> (seconds since 1Jan1904=w443:timestamp)
            n99 = while {
              shift-right: [w450] -> w444
              shift-left: w446 -> [w461]
              tunnel: w445 -> [w462]
              tunnel: w443 -> [w458]
              shift-right: [w448] -> _
              shift-left: w443 -> [w459]
              tunnel: [w457] -> _
              shift-right: [w449] -> _
              shift-left: w443 -> [w447]
              stop <- "End Collecting" stop-if-true
              n100 = call "Fetch&Process_Measurements.vi"("Rolling Timer Input"=w459, "error in (no error)"=w461, "Initial Time"=w458, "DCPowerInformation_byChannel"=w462, "Queue Data Parameters in"=T14 {"Rolling Timer"=timestamp(0 s since 1904-01-01), "Initial Time"=timestamp(0 s since 1904-01-01), "dt between samples"=[], "number of samples per fetch"=[], "voltage measurements"=[], "current measurements"=[]} ("Queue Data Parameters")) -> ("error out"=w451:errorcluster, "Current Measurement"=→"Current":waveform(dbl)[], "Voltage Measurement"=→"Voltage":waveform(dbl)[], "Queue Data Parameters out"=w457:T14, "Rolling Timer Output"=w448:timestamp)  [unwired: 2 in]
              n101 = Subtract(x=w448, y=w447) -> (x-y=w453:dbl)
              n102 = Greater?(x=w453, y=10.0) -> (0:w452:bool)
              n103 = disable-structure shown="Enabled" {
                disable-tunnel: w452 -> [w469 _]
                disable-tunnel: w451 -> [w468 w482]
                disable-tunnel: [w467 w482] -> w450
                disable-tunnel: [w466 w481] -> w449
                disable-tunnel: w448 -> [w465 w481]
                disable-tunnel: w447 -> [w464 _]
                frame Enabled {
                  n104 = case shown="True" w469 {
                    tunnel: w468 -> [w471 w480]
                    tunnel: [w471 w478] -> w467
                    tunnel: [w470 w472] -> w466
                    tunnel: w465 -> [_ w472]
                    tunnel: w464 -> [w470 _]
                    frame False {
                    }
                    frame True {
                      w475 = u8 0 ("X Scale.Scale Fit")
                      w476 = waveform(dbl)[][] [] ("History Data")
                      n105 = To Double Precision Float(number=w472) -> (double precision float=w473:dbl)
                      n106 = Add(x=w473, y=10.0) -> (x+y=w474:dbl)
                      n107 = property on="Voltage" class="WFChart (strict)"(error in=w480, "History Data"=w476, "XScale.ScaleFit"=w475, "XScale.Minimum"=w473, "XScale.Maximum"=w474) -> (error out=w479:errorcluster)  [unwired: 1 in, 1 out]
                      n108 = property on="Current" class="WFChart (strict)"(error in=w479, "History Data"=w476, "XScale.ScaleFit"=w475, "XScale.Minimum"=w473, "XScale.Maximum"=w474) -> (error out=w478:errorcluster)  [unwired: 1 in, 1 out]
                    }
                  }
                }
                frame Disabled {
                }
              }
            }
          }
          frame Enabled {
          }
        }
        n109 = for {
          tunnel: w400 -> [w429] mode=indexing
          tunnel: [w422] -> w391 mode=indexing
          tunnel: [w421] -> w390 mode=indexing
          tunnel: [w409] -> w387 mode=indexing
          tunnel: [w410] -> w385 mode=indexing
          tunnel: [w411] -> w386 mode=indexing
          tunnel: [w407] -> w384 mode=indexing
          tunnel: [w408] -> w388 mode=indexing
          shift-right: [w420] -> w393
          shift-left: w397 -> [w426]
          tunnel: w383 -> [w406]
          tunnel: [w405] -> w382 mode=indexing
          tunnel: [w404] -> w381 mode=indexing
          n110 = Unbundle(w429) -> ("IVI Refnum out"=w425:refnum<k15>, w428:string, "Channel Name 23"=w404:string, "Measure Record dt"=w408:dbl)  [unwired: 5 out]
          n111 = property class="niDCPower"(reference=w425, error in=w426, "Active Channel"=w428) -> (reference out=w424:refnum<k15>, error out=w423:errorcluster, "Fetch Backlog"=w427:i32)
          n112 = call <instrlib>:"niDCPower Fetch Multiple.vi"("instrument handle"=w424, "channel name"=w428, "count (1)"=w427, "error in (no error)"=w423) -> ("actual count"=w409:i32, "voltage measurements"=w411:dbl[], "current measurements"=w410:dbl[], "error out"=w420:errorcluster)  [unwired: 6 in, 2 out]
          n113 = Get Date/Time In Seconds() -> (seconds since 1Jan1904=w407:timestamp)
          n114 = Bundle By Name("Y"=w411, "dt"=w408, "t0"=w407) -> (w422:waveform(dbl))  [unwired: 1 out]
          n115 = Bundle By Name("Y"=w410, "dt"=w408, "t0"=w407) -> (w421:waveform(dbl))  [unwired: 1 out]
          n116 = To Double Precision Float(number=w407) -> (double precision float=w417:dbl)
          n117 = To Double Precision Float(number=w406) -> (double precision float=w416:dbl)
          n118 = call-poly <vilib>:"Ramp Pattern.vi"("start"=1.0, "end"=w409, "delta"=1.0) -> ("Ramp Pattern"=w413:dbl[])  [unwired: 6 in, 2 out]
          n119 = Multiply(x=w408, y=w413) -> (x*y=w412:dbl[])
          n120 = Subtract(x=w417, y=w416) -> (x-y=w414:dbl)
          n121 = Add(x=w414, y=w412) -> (x+y=w419:dbl[])
          n122 = Build Array(w419, w411, w410) -> (w405:dbl[][])
        }
        "Array" <- w382
        n123 = Bundle(w384, "seconds since 1Jan1904"=w383, w388, w387, "voltage measurements"=w386, "current measurements"=w385) -> (→"output cluster 2":T5)  [unwired: 1 in]
        n124 = Bundle(cluster=w380, "Array of fetched data"=w382, "Channel Names Array"=w381) -> (w379:T4)  [unwired: 4 in]
        n125 = Enqueue Element(queue=w394, element=w379, error in (no error)=w393) -> (error out=w389:errorcluster)  [unwired: 1 in, 2 out]
      }
    }
    "Voltage 2" <- w276
    "Current 2" <- w277
    n126 = And(x=w273, y=w272) -> (x .and. y?=w271:bool)
    n127 = case shown="True" w271 {
      tunnel: w270 -> [w296 w298]
      tunnel: [w297 TRUE] -> w254
      tunnel: w259 -> [w297 _]
      tunnel: [w296 w298] -> w265
      frame False {
      }
      frame True {
      }
    }
    "error of collection" <- w265
    "Ready For Next Run?" <- w254
    n128 = Or(x=w265, y="force exit SubVI") -> (x .or. y?=w267:bool)
    n129 = And(x="Next Run", y=w254) -> (x .and. y?=w269:bool)
    n130 = Or(x=w267, y=w269) -> (x .or. y?=w268:bool)
    n131 = case shown="True" w268 {
      selector: w268 -> [w287 _]
      tunnel: w267 -> [_ w290]
      tunnel: [w287 TRUE] -> w253
      tunnel: [TRUE ("T button?") w288] -> w263
      frame False {
        # "Don't end the run"
      }
      frame True {
        n132 = case shown="False" w290 {
          tunnel: [w291 TRUE] -> w288
          frame False {
            # "Option to continue the run as is or reset for a new configuration"
            n133 = Two Button Dialog(message="Would you like to change parameters before the next run? ( you will have an option to change LET and board number regardless) ", 1:"No, I may only want to change LET or board number" ("F button name (\"Cancel\")"), 2:"Yes, I want to make changes " ("T button name (\"OK\")")) -> (T button?=w291:bool)
          }
          frame True {
            # "End the run immediately. There is an error or an immediate issue with the VI"
          }
        }
      }
    }
    "Exiting" <- w253
  }
  "DCPowerInformationClusterArray_Output" <- w55
  "VISAPowerInfoInputOutput" <- w54
  "Run Data SubPanel Output" <- w53
  "RF Block Parameters Output" <- w52
  "Oscilloscope Info Array Output" <- w51
  "Reinitialize?" <- w44
  "Data Was Collected?" <- w21
  n134 = for {
    tunnel: w7 -> [w488] mode=indexing
    tunnel: w6 -> [w486] mode=indexing
    shift-right: [w484] -> w4
    shift-left: w5 -> [w487]
    n135 = Close File(refnum=w488, error in=w487) -> (error out=w485:errorcluster)  [unwired: 1 out]
    n136 = Close File(refnum=w486, error in=w485) -> (error out=w484:errorcluster)  [unwired: 1 out]
  }
  n137 = Merge Errors(w10, w4) -> (w3:errorcluster)
  n138 = disable-structure shown="Enabled" {
    disable-tunnel: w3 -> [w506 w556]
    disable-tunnel: w2 -> [w503 w557]
    disable-tunnel: [w489 w540] -> w1
    frame Disabled {
      w490 = 24
      (unwired) T4[] []
      # "structure where the instruments channels are all read in one file together"
      # "number of data file nodes"
      # "To be removed once we only have one data file node and one supplemental data file node channel again soon"
      n139 = List Folder(path=w503, error in=w506) -> (path out=w498:path, filenames=w505:string[], error out=w497:errorcluster)  [unwired: 2 in, 1 out]
      n140 = Array Size(array=w505) -> (size(s)=w504:i32)
      n141 = Multiply(x=w490, y=2) -> (x*y=w500:i32)
      n142 = Divide(x=w504, y=w500) -> (x/y=w502:dbl)
      n143 = Decrement(x=w502) -> (x-1=w501:dbl)
      n144 = for {
        N: w501 -> [_]
        tunnel: w498 -> [w527]
        shift-right: [w523] -> w489
        shift-left: w497 -> [w525]
        tunnel: T4 {"Array of fetched data"=[], "Channel Names Array"=[], "Voltage Waveform Array"=[], "Current Waveform Array"=[], "Resetting Time"=timestamp(0 s since 1904-01-01), "Beam Logic"=0.0} ("DCPower Queue Data Double Array Format") -> [w514]
        tunnel: [w508] -> w491 mode=concatenating
        tunnel: [w508] -> w495 mode=indexing
        tunnel: [w511] -> w494 mode=indexing
        tunnel: [w511] -> w493 mode=concatenating
        tunnel: 0 ("size(s)") -> [w510]
        tunnel: w490 -> [w509]
        i -> [w534]
        w515 = T16."open" ("operation (0:open)")
        w532 = "NULL0_part_"
        # "Will need to change the naming conventions for this"
        n145 = Increment(x=w534) -> (x+1=w535:i32)
        n146 = Number To Decimal String(number=w535) -> (decimal integer string=w531:string)  [unwired: 1 in]
        n147 = Concatenate Strings(w532, w531, "_datafile.bin") -> (w529:string)
        n148 = Concatenate Strings(w532, w531, "_supplementaldatanode.bin") -> (w528:string)
        n149 = Build Path(base path=w527, name or relative path=w529) -> (appended path=w526:path)
        n150 = Build Path(base path=w527, name or relative path=w528) -> (appended path=w524:path)
        n151 = Open/Create/Replace File(file path (use dialog)=w526, error in=w525, operation (0:open)=w515) -> (refnum out=w518:refnum<file>, error out=w519:errorcluster)  [unwired: 3 in, 1 out]
        n152 = Read from Binary File(5:w514, 8:w519, 9:T15."native, host order" ("byte order (0:big-endian, network order)"), 10:-1 ("count (1)"), 11:w518) -> (0:w520:errorcluster, 2:w508:T4[])  [unwired: 1 in, 2 out]
        "datafile in loop" <- w508
        n153 = Open/Create/Replace File(file path (use dialog)=w524, error in=w520, operation (0:open)=w515) -> (refnum out=w521:refnum<file>, error out=w522:errorcluster)  [unwired: 3 in, 1 out]
        n154 = Read from Binary File(5:w510, 8:w522, 9:T15."native, host order" ("byte order (0:big-endian, network order)"), 10:-1 ("count (1)"), 11:w521) -> (0:w523:errorcluster, 2:w511:i32[])  [unwired: 1 in, 2 out]
        "supplemental datafile" <- w511
        n155 = for {
          tunnel: w508 -> [w536]
          i -> [w537]
          n156 = Index Array(array=w536, index=w537) -> ()  [unwired: 1 out]
        }
      }
      "datafile in concatenation" <- w491
      "datafile in array" <- w495
      "supplemental datafile array" <- w494
      "supplemental datafile concatenated" <- w493
      n157 = for {
        tunnel: w491 -> [w507] mode=indexing
      }
    }
    frame Enabled {
      # "number of bin files"
      # "datafile and supplemental parameters file"
      # "for now it will be 24 since we're using all channells of a 4163"
      # "NEED DATA PARAMETERS FILE TO KNOW HOW MANY DC POWER LOGS WERE RECORDED TO ACCURATELY PARSE THIS"
      n158 = List Folder(path=w557, error in=w556) -> (path out=w546:path, filenames=w555:string[], error out=w549:errorcluster)  [unwired: 2 in, 1 out]
      n159 = Array Size(array=w555) -> (size(s)=w554:i32)
      n160 = Multiply(x=24.0, y=2.0) -> (x*y=w551:dbl)
      n161 = Divide(x=w554, y=w551) -> (x/y=w539:dbl)
      n162 = Decrement(x=w539) -> (x-1=w538:dbl)
      n163 = for {
        tunnel: w546 -> [w586]
        tunnel: string[] ["NULL0", "NULL1", "NULL2", "NULL3", "NULL4", "NULL5", "NULL6", "NULL7", "NULL8", "NULL9", "NULL10", "NULL11", "NULL12", "NULL13", "NULL14", "NULL15", "NULL16", "NULL17", "NULL18", "NULL19", "NULL20", "NULL21", "NULL22", "NULL23"] -> [w587] mode=indexing
        tunnel: w538 -> [w583]
        shift-right: [w585] -> w545
        shift-left: w549 -> [w584]
        tunnel: T3 {"Array of fetched data"=[], "", []} ("output cluster") -> [w582]
        tunnel: [w581] -> w547 mode=indexing
        n164 = for {
          N: w583 -> [_]
          tunnel: w587 -> [w608]
          tunnel: w586 -> [w602]
          shift-right: [w598] -> w585
          shift-left: w584 -> [w601]
          tunnel: w582 -> [w600]
          tunnel: [w596] -> w581 mode=concatenating
          i -> [w589]
          n165 = Increment(x=w589) -> (x+1=w588:i32)
          n166 = Number To Decimal String(number=w588) -> (decimal integer string=w610:string)  [unwired: 1 in]
          n167 = Concatenate Strings(w608, "_part_" ("string"), w610, "_datafile.bin" ("string")) -> (w603:string)
          n168 = Build Path(base path=w602, name or relative path=w603) -> (appended path=w605:path)
          n169 = Open/Create/Replace File(file path (use dialog)=w605, error in=w601, operation (0:open)=T16."open", access (0:read/write)=enum16{"read/write", "read-only", "write-only"}."read/write") -> (refnum out=w594:refnum<file>, error out=w595:errorcluster)  [unwired: 2 in, 1 out]
          n170 = Set File Position(refnum=w594, error in=w595) -> (refnum out=w593:refnum<file>, error out=w592:errorcluster)  [unwired: 2 in]
          n171 = Read from Binary File(5:w600, 8:w592, 9:T15."native, host order" ("byte order (0:big-endian, network order)"), 10:-1 ("count (1)"), 11:w593) -> (0:w599:errorcluster, 2:w596:T2, 3:w597:refnum<file>)  [unwired: 1 in, 1 out]
          "data iterating in loop" <- w596
          n172 = Close File(refnum=w597, error in=w599) -> (error out=w598:errorcluster)  [unwired: 1 out]
        }
        "each channel cluster" <- w581
      }
      "all channel clusters as a large array" <- w547
      n173 = for {
        tunnel: w547 -> [w576] mode=indexing
        tunnel: [w567] -> w544 mode=indexing
        tunnel: w546 -> [w571]
        shift-right: [w573] -> w541
        shift-left: w545 -> [w575]
        n174 = for {
          tunnel: w576 -> [w580] mode=indexing
          tunnel: [w579] -> w567 mode=concatenating
          shift-right: [w578] -> w574
          shift-left: w575 -> [w578]
          tunnel: [w577] -> w569 mode=indexing
          n175 = Unbundle(w580) -> ("Array of fetched data"=w579:dbl[][], w577:string)  [unwired: 1 out]
        }
        n176 = Concatenate Strings(w569, "_output.csv" ("string")) -> (w570:string)
        n177 = Build Path(base path=w571, name or relative path=w570) -> (appended path=w572:path)
        n178 = call-poly <vilib>:"Write Delimited Spreadsheet.vi"("file path (dialog if empty)"=w572, "2D data"=w567, "error in (no error)"=w574) -> ("error out"=w573:errorcluster)  [unwired: 11 in, 1 out]
      }
      n179 = for {
        tunnel: w544 -> [w561] mode=indexing
        shift-right: [w560] -> w542
        shift-left: dbl[][] [] ("Array of fetched data") -> [w562]
        shift-right: [w558] -> w540
        shift-left: w541 -> [w559]
        n180 = for {
          tunnel: w561 -> [w565] mode=indexing
          shift-right: [w564] -> w560
          shift-left: w562 -> [w566]
          shift-right: [w563] -> w558
          shift-left: w559 -> [w563]
          n181 = Insert Into Array(array=w566, new element=w565) -> (w564:dbl[][])  [unwired: 2 in]
        }
      }
      "Array of all channels?" <- w542
    }
  }
  "error out" <- w1
